vi "Write States.vi"(8 "error in (no error)":errorcluster, 10 "States":enum16{"PenaltyPos", "Exit"}(ring), 11 "PenaltyAttackTacticVSS in":refnum<class "PenaltyAttackTacticVSS.lvclass">) -> (0 "error out":errorcluster, 3 "PenaltyAttackTacticVSS out":refnum<class "PenaltyAttackTacticVSS.lvclass">)   [LabVIEW 2018, in "PenaltyAttackTacticVSS.lvclass"]
uses:
  PenaltyAttackTacticVSS.lvclass
  PenaltyAttackTacticVSS.lvclass/PenaltyAttackTacticVSS.ctl
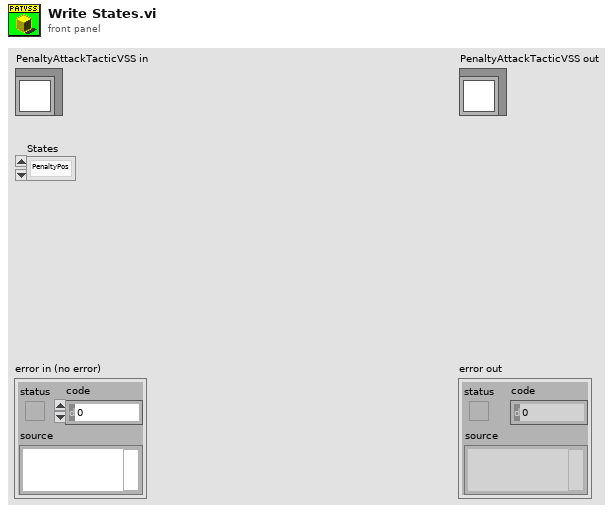
[diagram p1: front panel]
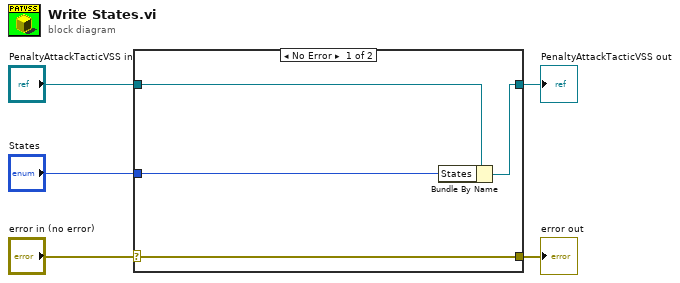
[diagram p0: block diagram]
diagram:
  n1 = case shown="No Error" "error in (no error)" {
    selector: "error in (no error)" -> [w9 w10]
    tunnel: [w9 w10] -> w4
    tunnel: [w7 w11] -> w2
    tunnel: "PenaltyAttackTacticVSS in" -> [w8 w11]
    tunnel: "States" -> [w6 _]
    frame No Error {
      n2 = Bundle By Name(cluster=w8, "States"=w6) -> (w7:refnum<class "PenaltyAttackTacticVSS.lvclass">)
    }
    frame Error {
    }
  }
  "error out" <- w4
  "PenaltyAttackTacticVSS out" <- w2
